vi "RANGE Auto Mode.vi"(4 "Meter 246":string="A", 5 "SLPM Error @ Zero (2,4,6)":dbl, 6 "Meter 135":string="A", 7 "SLPM Error @ Zero (1,3,5)":dbl, 8 "Error In":errorcluster, 10 "Meter 2,4,6":T1, 11 "Meter 1,3,5":T1) -> (0 "Error Out":errorcluster, 1 "Meter ID":string, 2 "Status":string, 3 "Output":T1)   [LabVIEW 2016]
uses:
  Drivers/Alicat Gas Meter Driver/Sub-VIs/Data Cluster.ctl
panel:
  # "Totalizer Timer"
  # "Totalizer Timer"
  # "Totalizer Timer"
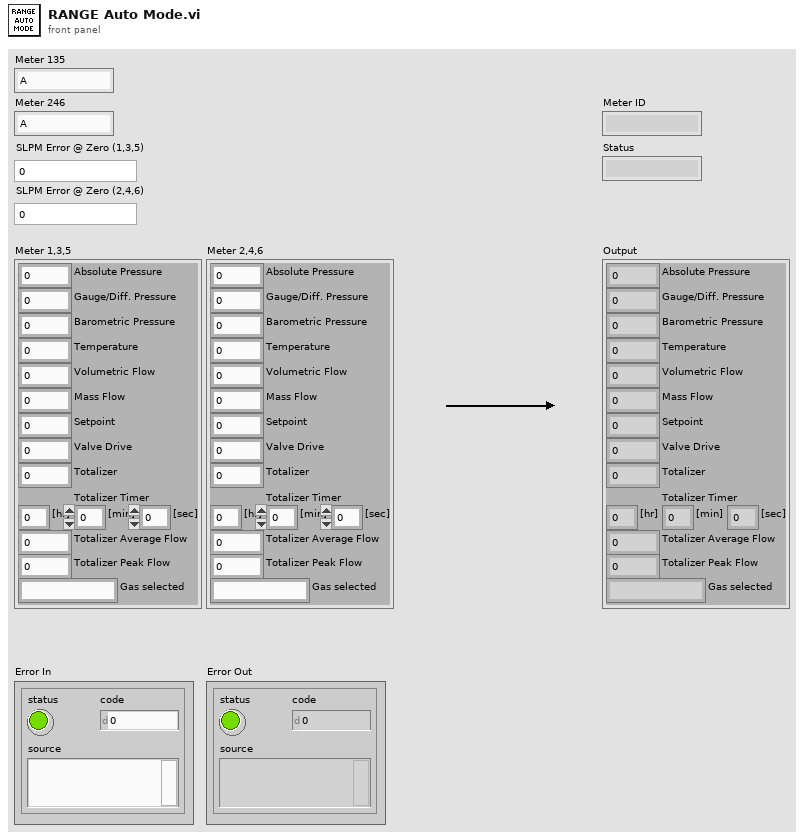
[diagram p1: front panel]
types:
  T1 = typedef "Data Cluster.ctl" = cluster{"Absolute Pressure":dbl, "Gauge/Diff. Pressure":dbl, "Barometric Pressure":dbl, "Temperature":dbl, "Volumetric Flow":dbl, "Mass Flow":dbl, "Setpoint":dbl, "Valve Drive":dbl, "Totalizer":dbl, "[hr]":dbl, "[min]":dbl, "[sec]":dbl, "Totalizer Average Flow":dbl, "Totalizer Peak Flow":dbl, "Gas selected":string}
  T2 = cluster{"Absolute Pressure":dbl, "Gauge/Diff. Pressure":dbl, "Barometric Pressure":dbl, "Temperature":dbl, "Volumetric Flow":dbl, "Mass Flow":dbl, "Setpoint":dbl, "Valve Drive":dbl, "Totalizer":dbl, "[hr]":dbl, "[min]":dbl, "[sec]":dbl, "Totalizer Average Flow":dbl, "Totalizer Peak Flow":dbl, "Gas selected":string}
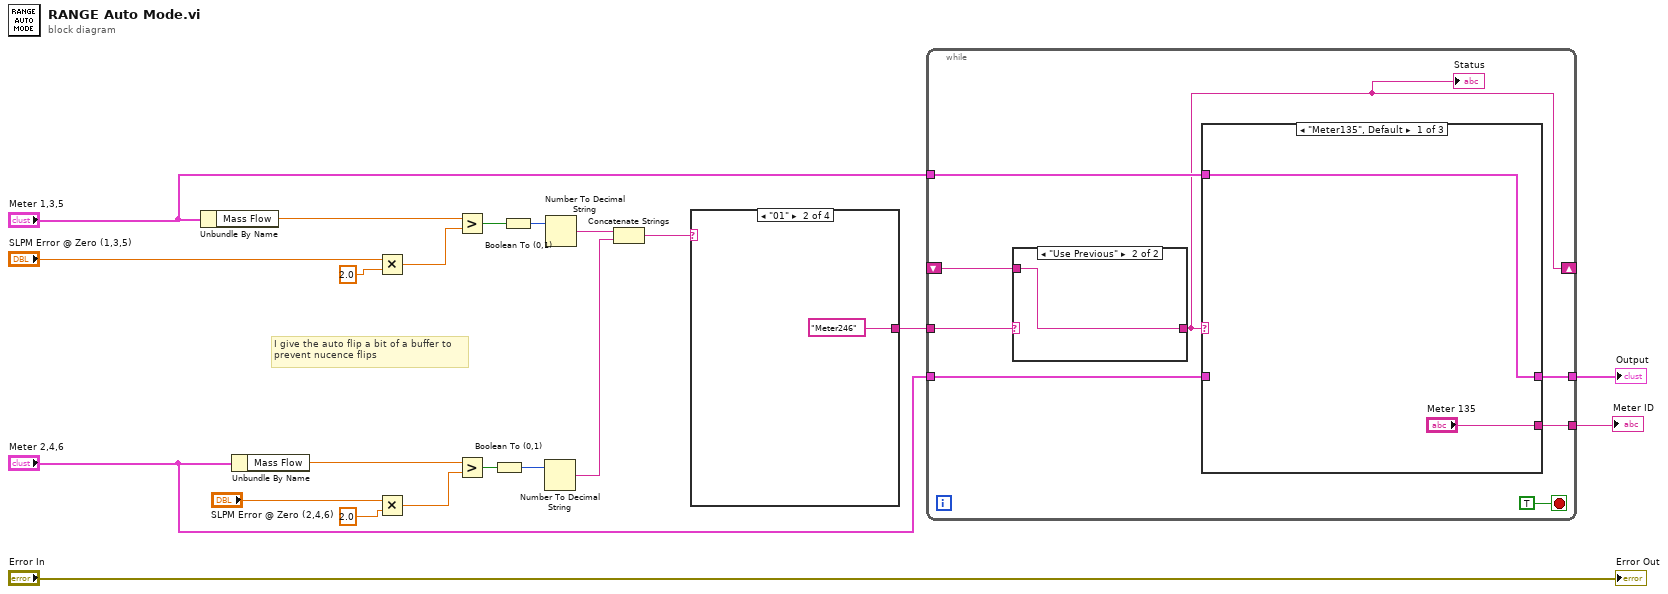
[diagram p0: block diagram]
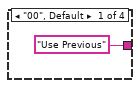
[diagram p2: hidden frame]
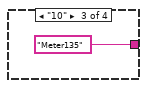
[diagram p3: hidden frame]
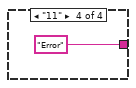
[diagram p4: hidden frame]
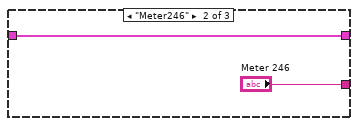
[diagram p6: hidden frame]
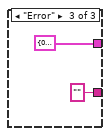
[diagram p7: hidden frame]
diagram:
  # "I give the auto flip a bit of a buffer to\nprevent nucence flips"
  n1 = Unbundle By Name("Meter 1,3,5") -> ("Mass Flow"=w5:dbl)
  n2 = Unbundle By Name("Meter 2,4,6") -> ("Mass Flow"=w15:dbl)
  n3 = Multiply(x="SLPM Error @ Zero (1,3,5)", y=2.0) -> (x*y=w16:dbl)
  n4 = Multiply(x="SLPM Error @ Zero (2,4,6)", y=2.0) -> (x*y=w14:dbl)
  n5 = Greater?(x=w5, y=w16) -> (0:w13:bool)
  n6 = Greater?(x=w15, y=w14) -> (0:w12:bool)
  n7 = Boolean To (0,1)(Boolean=w12) -> (0, 1=w10:i16)
  n8 = Boolean To (0,1)(Boolean=w13) -> (0, 1=w11:i16)
  n9 = Number To Decimal String(number=w10) -> (decimal integer string=w8:string)  [unwired: 1 in]
  n10 = Number To Decimal String(number=w11) -> (decimal integer string=w9:string)  [unwired: 1 in]
  n11 = Concatenate Strings(w9, w8) -> (w7:string)
  n12 = case shown="\"01\"" w7 {
    tunnel: ["Use Previous" "Meter246" "Meter135" "Error"] -> w6
    frame "00", Default {
    }
    frame "01" {
    }
    frame "10" {
    }
    frame "11" {
    }
  }
  n13 = while {
    tunnel: "Meter 1,3,5" -> [w33]
    tunnel: [w31] -> w2
    tunnel: "Meter 2,4,6" -> [w30]
    shift-right: [w27] -> _
    shift-left: _ -> [w29]
    tunnel: w6 -> [w28]
    tunnel: [w26] -> w1
    stop <- TRUE stop-if-true
    n14 = case shown="\"Use Previous\"" w28 {
      selector: w28 -> [w34 _]
      tunnel: w29 -> [_ w35]
      tunnel: [w34 w35] -> w27
      frame Default {
      }
      frame "Use Previous" {
      }
    }
    "Status" <- w27
    n15 = case shown="\"Meter135\", Default" w27 {
      tunnel: w33 -> [w37 _ _]
      tunnel: [w37 w39 T2 {"Absolute Pressure"=0.0, "Gauge/Diff. Pressure"=0.0, "Barometric Pressure"=0.0, "Temperature"=0.0, "Volumetric Flow"=0.0, "Mass Flow"=0.0, "Setpoint"=0.0, "Valve Drive"=0.0, "Totalizer"=0.0, "[hr]"=0.0, "[min]"=0.0, "[sec]"=0.0, "Totalizer Average Flow"=0.0, "Totalizer Peak Flow"=0.0, "Gas selected"=""} ("Meter 2,4,6")] -> w31
      tunnel: w30 -> [_ w39 _]
      tunnel: ["Meter 135" "Meter 246" "" ("Meter 246")] -> w26
      frame "Meter135", Default {
      }
      frame "Meter246" {
      }
      frame "Error" {
      }
    }
  }
  "Output" <- w2
  "Meter ID" <- w1
  "Error Out" <- "Error In"
